vi "Test Arduino.vi"() -> ()   [LabVIEW 2023, in "Arduino DAQ.lvlib"]
uses:
  Arduino DAQ.lvlib
  <vilib>/Instr/_visa.llb/VISA Configure Serial Port (Instr).vi
panel:
  out "Startup Message":string
  out "OK?":bool
  in  "VISA resource name":refnum<visa-resource-name>="COM3"
  out "error out":errorcluster
  in  "error in (no error)":errorcluster
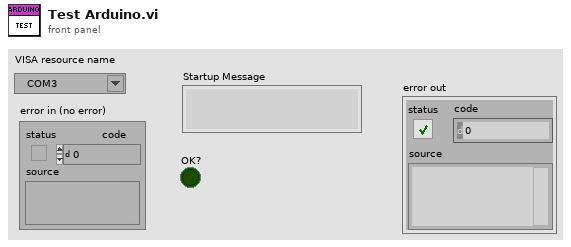
[diagram p1: front panel]
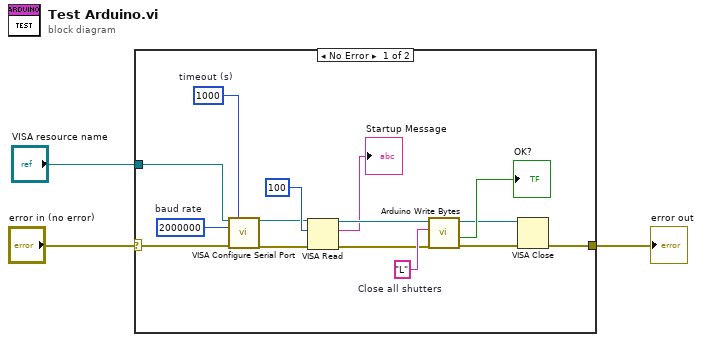
[diagram p0: block diagram]
diagram:
  n1 = case shown="No Error" "error in (no error)" {
    selector: "error in (no error)" -> [w17 w19]
    tunnel: [w10 w19] -> w3
    tunnel: "VISA resource name" -> [w15 _]
    frame No Error {
      w14 = "L"  # Close all shutters
      w16 = u32 1000  # timeout (s)
      w18 = u32 2000000  # baud rate
      n2 = call-poly "VISA Configure Serial Port"("VISA resource name"=w15, "timeout (10sec)"=w16, "baud rate (9600)"=w18, "error in (no error)"=w17) -> ("VISA resource name out"=w7:refnum<visa-resource-name>, "error out"=w8:errorcluster)  [unwired: 10 in]
      n3 = VISA Read(VISA resource name=w7, byte count=u32 100, error in (no error)=w8) -> (VISA resource name out=w5:refnum<visa-resource-name>, read buffer=→"Startup Message":string, error out=w6:errorcluster)  [unwired: 1 out]
      n4 = call "Arduino Write Bytes.vi"("error in (no error)"=w6, "Command"=w14, "COM Port In"=w5) -> ("error out"=w11:errorcluster, "OK?"=→"OK?":bool, "COM Port Out"=w12:refnum<visa-resource-name>)  [unwired: 5 in, 1 out]
      n5 = VISA Close(VISA resource name=w12, error in (no error)=w11) -> (error out=w10:errorcluster)
    }
    frame Error {
    }
  }
  "error out" <- w3
